vi "fridge night watcher.vi"() -> ()   [LabVIEW 2010]
uses:
  <userlib>/Nanonis Prog Interface V5/Nanonis Prog Interface.lvlib
panel:
  out "Response":string
  out "Loops":i32
  out "State":enum16{"START", "LOWER", "HIGHER", "STALL"}(ring)
  in  "Current Upper Limit":dbl=2.6
  in  "Current Lower Limit":dbl=1.8
  out "Not Stalled?":bool
  in  "Higher Voltage":dbl=9.8
  in  "Lower Voltage":dbl=3.5
  out "Current RMS (pA)":sgl format="%#_6p"
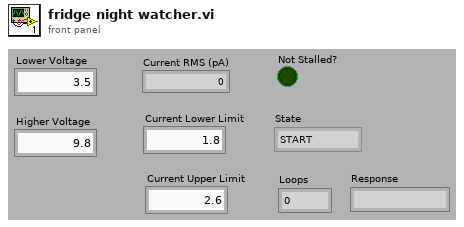
[diagram p1: front panel]
types:
  T1 = enum16{"Set Heater Voltage", "Read Heater Voltage", "Read Heater Current", "Read 1K Pot Temperature", "Read IVC Sorb Temperature", "Read Needle Valve Temperature", "Read Still Pressure", "Read Mixing Chamber Temperature", "Read STM RX Temperature", "Read STM CX Temperature", "Unstall Triton Loop", "Triton Stop", "Triton Stall Status"}
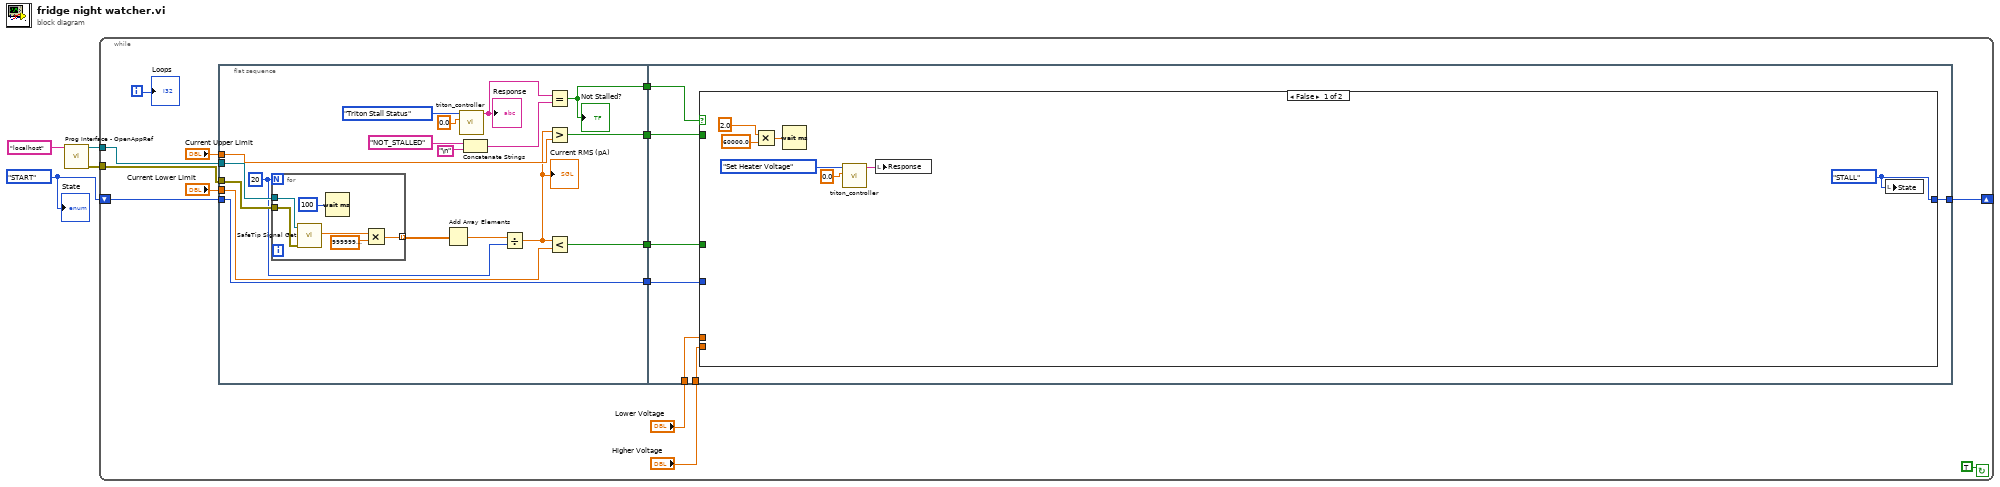
[diagram p0: block diagram]
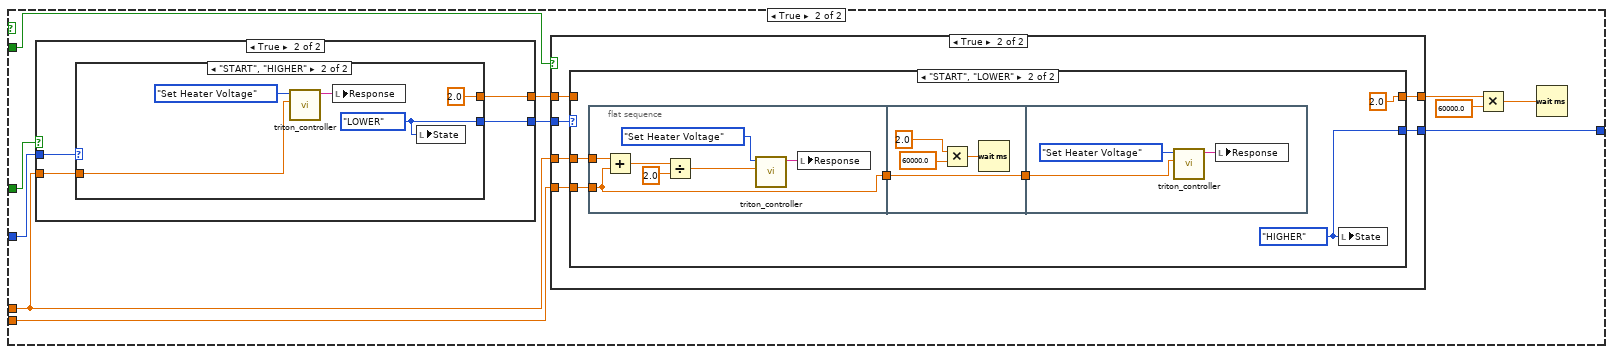
[diagram p2: hidden frame]
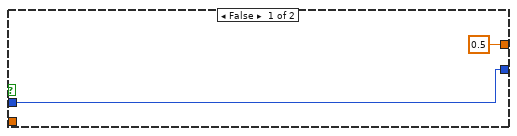
[diagram p5: hidden frame]
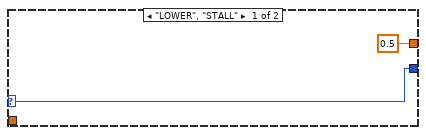
[diagram p6: hidden frame]
diagram:
  w1 = enum16{"START", "LOWER", "HIGHER", "STALL"}."START" ("Enum")
  n1 = call <userlib>:"Prog Interface - OpenAppRef.vi"("Machine name (local machine IP)"="localhost" ("machine name (localhost)")) -> ("Error out"=w2:errorcluster, "Application reference"=w3:refnum<vi>)  [unwired: 5 in]
  n2 = while {
    tunnel: w3 -> [w15]
    tunnel: w2 -> [w14]
    shift-right: [w10] -> _
    shift-left: w1 -> [w12]
    i -> [w9]
    stop <- TRUE continue-if-true
    n3 = flat-sequence {
      tunnel: w15 -> [w36]
      tunnel: w14 -> [w35]
      tunnel: [w25] -> w18
      tunnel: "Current Lower Limit" -> [w24]
      tunnel: [w23] -> w17
      tunnel: "Current Upper Limit" -> [w22]
      tunnel: [w20] -> w16
      tunnel: w12 -> [w19]
      tunnel: [w19] -> w11
      tunnel: w18 -> [w49]
      tunnel: w17 -> [w48]
      tunnel: w16 -> [w47]
      tunnel: "Lower Voltage" -> [w46]
      tunnel: "Higher Voltage" -> [w45]
      tunnel: w11 -> [w44]
      tunnel: [w43] -> w10
      frame #0 {
        w32 = 20
        n4 = for {
          N: w32 -> [_]
          tunnel: w36 -> [w42]
          tunnel: w35 -> [w41]
          tunnel: [w37] -> w34 mode=indexing
          n5 = call <userlib>:"SafeTip Signal Get.vi"("error in (no error)"=w41, "Application ref in"=w42) -> ("SafeTip signal value"=w40:sgl)  [unwired: 7 in, 2 out]
          n6 = Wait (ms)(milliseconds to wait=u32 100) -> ()  [unwired: 1 out]
          n7 = Multiply(x=w40, y=sgl 1000000000000.0) -> (x*y=w37:sgl)
        }
        n8 = Add Array Elements(numeric array=w34) -> (sum=w33:sgl)
        n9 = call "triton_controller.vi"("Numerical Argument"=0.0, "Command"=T1."Triton Stall Status") -> ("Response"=w29:string)  [unwired: 9 in]
        "Response" <- w29
        n10 = Concatenate Strings("NOT_STALLED" ("y"), "\n") -> (w28:string)
        n11 = Divide(x=w33, y=w32) -> (x/y=w21:sgl)
        "Current RMS (pA)" <- w21
        n12 = Equal?(x=w29, y=w28) -> (x = y?=w25:bool)
        "Not Stalled?" <- w25
        n13 = Greater?(x=w21, y=w22) -> (0:w20:bool)
        n14 = Less?(x=w21, y=w24) -> (x < y?=w23:bool)
      }
      frame #1 {
        n15 = case shown="False" w49 {
          tunnel: w48 -> [_ w67]
          tunnel: w47 -> [_ w66]
          tunnel: w46 -> [_ w57]
          tunnel: w45 -> [_ w65]
          tunnel: w44 -> [_ w64]
          tunnel: [w51 w62] -> w43
          frame False {
            w51 = enum16{"START", "LOWER", "HIGHER", "STALL"}."STALL" ("Enum")
            n16 = Multiply(x=2.0, y=60000.0) -> (x*y=w52:dbl)
            n17 = Wait (ms)(milliseconds to wait=w52) -> ()  [unwired: 1 out]
            n18 = call "triton_controller.vi"("Numerical Argument"=0.0, "Command"=T1."Set Heater Voltage") -> ("Response"=w50:string)  [unwired: 9 in]
            n19 = local write "Response"(w50) -> ()
            n20 = local write "State"(w51) -> ()
          }
          frame True {
            n21 = case shown="True" w67 {
              tunnel: w57 -> [_ w103]
              tunnel: w64 -> [w99 w102]
              tunnel: [w99 w101] -> w63
              tunnel: [0.5 ("x") w100] -> w59
              frame False {
              }
              frame True {
                n22 = case shown="\"START\", \"HIGHER\"" w102 {
                  selector: w102 -> [w105 _]
                  tunnel: w103 -> [_ w109]
                  tunnel: [w105 w107] -> w101
                  tunnel: [0.5 ("x") 2.0 ("x")] -> w100
                  frame "LOWER", "STALL" {
                  }
                  frame "START", "HIGHER" {
                    w107 = enum16{"START", "LOWER", "HIGHER", "STALL"}."LOWER" ("Enum")
                    n23 = call "triton_controller.vi"("Numerical Argument"=w109, "Command"=T1."Set Heater Voltage") -> ("Response"=w106:string)  [unwired: 9 in]
                    n24 = local write "Response"(w106) -> ()
                    n25 = local write "State"(w107) -> ()
                  }
                }
              }
            }
            n26 = case shown="True" w66 {
              tunnel: w65 -> [_ w75]
              tunnel: w63 -> [w69 w74]
              tunnel: [w69 w73] -> w62
              tunnel: w59 -> [w68 w72]
              tunnel: [w68 w71] -> w58
              tunnel: w57 -> [_ w70]
              frame False {
              }
              frame True {
                n27 = case shown="\"START\", \"LOWER\"" w74 {
                  selector: w74 -> [w77 _]
                  tunnel: w75 -> [_ w83]
                  tunnel: [w77 w81] -> w73
                  tunnel: [w76 2.0 ("x")] -> w71
                  tunnel: w72 -> [w76 _]
                  tunnel: w70 -> [_ w78]
                  frame "HIGHER", "STALL" {
                  }
                  frame "START", "LOWER" {
                    w81 = enum16{"START", "LOWER", "HIGHER", "STALL"}."HIGHER" ("Enum")
                    n28 = flat-sequence {
                      tunnel: w83 -> [w87]
                      tunnel: [w87] -> w79
                      tunnel: w78 -> [w88]
                      tunnel: [w94] -> w80
                      tunnel: w79 -> [w94]
                      tunnel: w80 -> [w96]
                      frame #0 {
                        n29 = Add(x=w88, y=w87) -> (x+y=w86:dbl)
                        n30 = Divide(x=w86, y=2.0) -> (x/y=w84:dbl)
                        n31 = call "triton_controller.vi"("Numerical Argument"=w84, "Command"=T1."Set Heater Voltage") -> ("Response"=w89:string)  [unwired: 9 in]
                        n32 = local write "Response"(w89) -> ()
                      }
                      frame #1 {
                        n33 = Multiply(x=2.0, y=60000.0) -> (x*y=w93:dbl)
                        n34 = Wait (ms)(milliseconds to wait=w93) -> ()  [unwired: 1 out]
                      }
                      frame #2 {
                        n35 = call "triton_controller.vi"("Numerical Argument"=w96, "Command"=T1."Set Heater Voltage") -> ("Response"=w95:string)  [unwired: 9 in]
                        n36 = local write "Response"(w95) -> ()
                      }
                    }
                    n37 = local write "State"(w81) -> ()
                  }
                }
              }
            }
            n38 = Multiply(x=w58, y=60000.0) -> (x*y=w60:dbl)
            n39 = Wait (ms)(milliseconds to wait=w60) -> ()  [unwired: 1 out]
          }
        }
      }
    }
    "Loops" <- w9
  }
  "State" <- w1
